vi "Write Type.vi"(8 "error in (no error)":errorcluster, 10 "Type":string, 11 "Instruction in":refnum<class "Instruction.lvclass">) -> (0 "error out":errorcluster, 3 "Instruction out":refnum<class "Instruction.lvclass">)   [LabVIEW 2015, in "Instruction.lvclass"]
uses:
  Instruction.lvclass
  Instruction.lvclass/Instruction.ctl
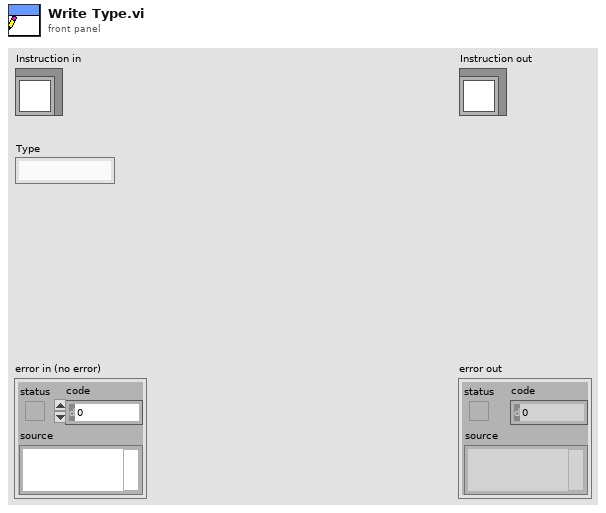
[diagram p1: front panel]
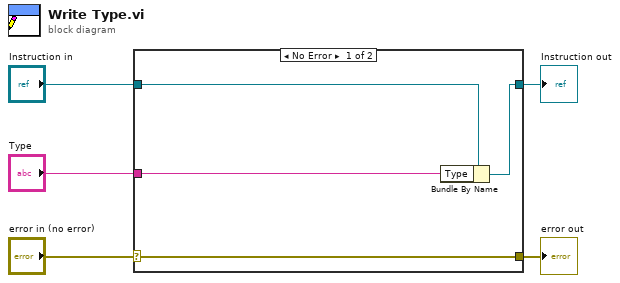
[diagram p0: block diagram]
diagram:
  n1 = case shown="No Error" "error in (no error)" {
    selector: "error in (no error)" -> [w9 w10]
    tunnel: [w9 w10] -> w4
    tunnel: [w7 w11] -> w2
    tunnel: "Instruction in" -> [w8 w11]
    tunnel: "Type" -> [w6 _]
    frame No Error {
      n2 = Bundle By Name(cluster=w8, "Type"=w6) -> (w7:refnum<class "Instruction.lvclass">)
    }
    frame Error {
    }
  }
  "error out" <- w4
  "Instruction out" <- w2
